vi "add logppms(SubVI).vi"(10 "字符串":string) -> (1 "ok or cancel":bool=TRUE, 2 "连接的字符串":string)   [LabVIEW 2019, in "SubVI.lvlib"]
uses:
  SubVI.lvlib
panel:
  in  "interval":dbl
  in  "cancel":bool
  in  "ok":bool
  in  "path":path
  in  "operation(0:open)":T1(ring)=enum."create"
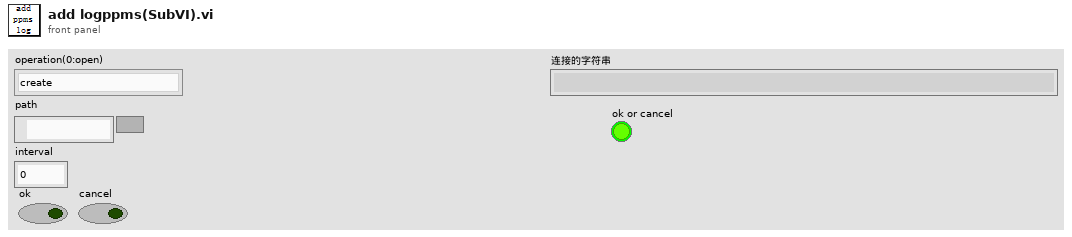
[diagram p1: front panel]
types:
  T1 = enum16{"open", "replace", "create", "open or create", "replace or create"}
  T2 = enum16{"open", "replace", "create", "open or create", "replace or create", "replace or create with confirmation"}
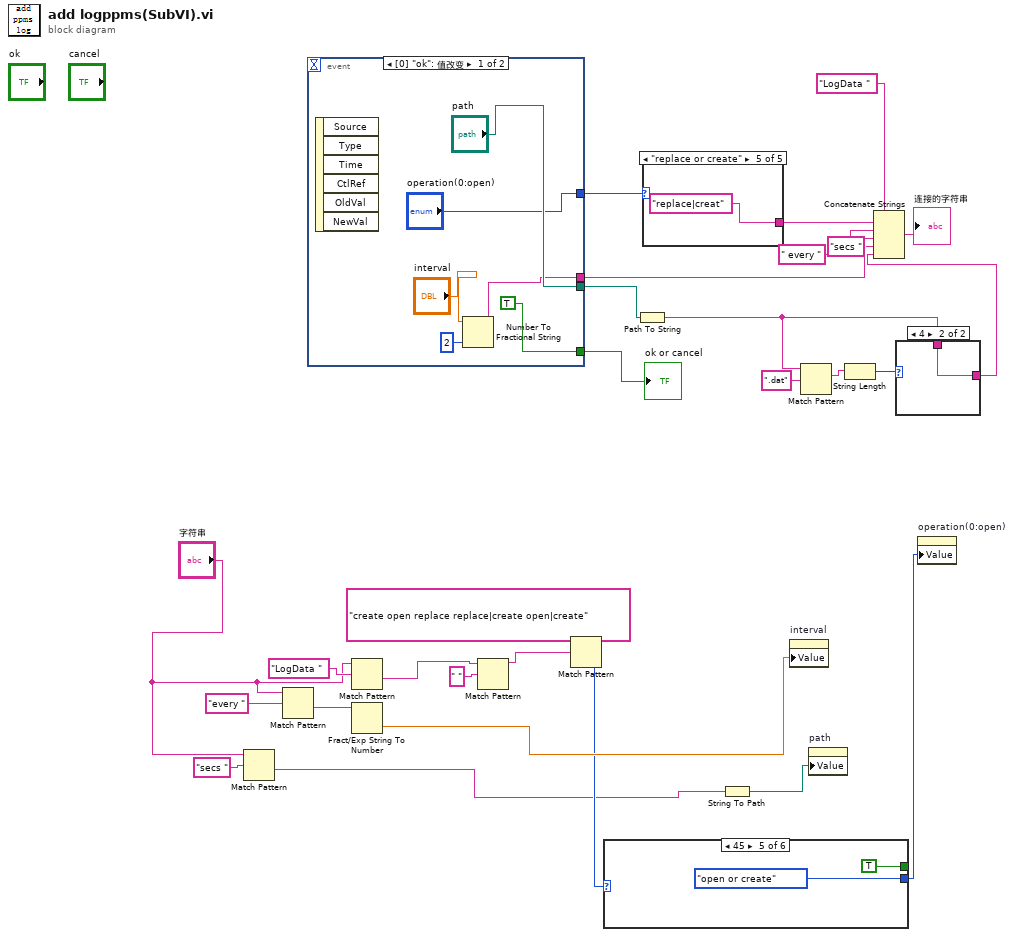
[diagram p0: block diagram]
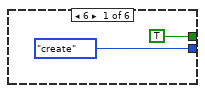
[diagram p2: hidden frame]
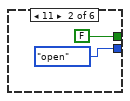
[diagram p3: hidden frame]
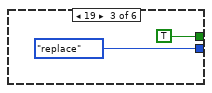
[diagram p4: hidden frame]
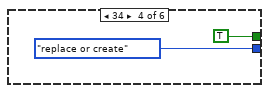
[diagram p5: hidden frame]
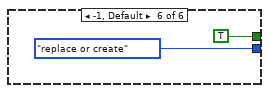
[diagram p6: hidden frame]
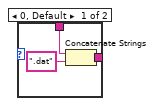
[diagram p7: hidden frame]
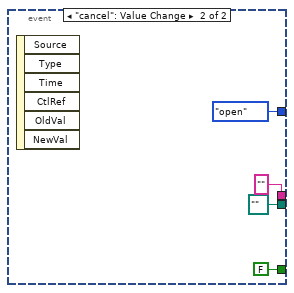
[diagram p8: hidden frame]
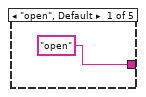
[diagram p9: hidden frame]
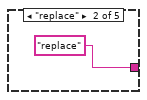
[diagram p10: hidden frame]
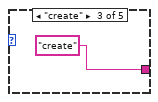
[diagram p11: hidden frame]
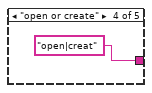
[diagram p12: hidden frame]
diagram:
  n1 = Match Pattern(string="字符串", regular expression="secs " ("正则表达式")) -> (after substring=w2:string)  [unwired: 1 in, 3 out]
  n2 = Match Pattern(string="字符串", regular expression="every " ("正则表达式")) -> (after substring=w11:string)  [unwired: 1 in, 3 out]
  n3 = event shown="[0] \"ok\": 值改变" {
    selector: _ -> [_ _]
    dyn-events: _ -> [_ _]
    timeout: _ -> [_ _]
    tunnel: ["path" path "" ("path")] -> w22
    tunnel: ["operation(0:open)" T1."open" ("operation(0:open)")] -> w27
    tunnel: [TRUE FALSE] -> w23
    tunnel: [w30 ""] -> w21
    event "ok": Value Change {
      n4 = event-data() -> ()  [unwired: 1 in, 6 out]
      n5 = Number To Fractional String(number="interval", precision (6)=i16 2 ("精度(6)")) -> (F-format string=w30:string)  [unwired: 2 in]
    }
    event "cancel": Value Change {
      n6 = event-data() -> ()  [unwired: 1 in, 6 out]
    }
  }
  "ok or cancel" <- w23
  n7 = Match Pattern(string="字符串", regular expression="LogData " ("正则表达式")) -> (after substring=w8:string)  [unwired: 1 in, 3 out]
  n8 = Fract/Exp String To Number(string=w11) -> (number=w5:dbl)  [unwired: 3 in, 1 out]
  n9 = Match Pattern(string=w8, regular expression=" " ("正则表达式")) -> (before substring=w7:string)  [unwired: 1 in, 3 out]
  n10 = Match Pattern(string="create open replace replace|create open|create" ("字符串"), regular expression=w7) -> (offset past match=w4:i32)  [unwired: 1 in, 3 out]
  n11 = case shown="45" w4 {
    tunnel: [T2."create" ("操作(0:open)") T2."open" ("操作(0:open)") T2."replace" ("操作(0:open)") T2."replace or create" ("操作(0:open)") T2."open or create" ("操作(0:open)") T2."replace or create" ("操作(0:open)")] -> w3
    tunnel: [TRUE FALSE TRUE TRUE TRUE TRUE] -> _
    frame 6 {
    }
    frame 11 {
    }
    frame 19 {
    }
    frame 34 {
    }
    frame 45 {
    }
    frame -1, Default {
    }
  }
  n12 = Path To String(path=w22) -> (string=w16:string)
  n13 = case shown="\"replace or create\"" w27 {
    tunnel: ["open" "replace" "create" "open|creat" "replace|creat"] -> w26
    frame "open", Default {
    }
    frame "replace" {
    }
    frame "create" {
    }
    frame "open or create" {
    }
    frame "replace or create" {
    }
  }
  n14 = String To Path(string=w2) -> (path=w1:path)
  n15 = property on="interval" class="DigNum (严格)"("Value"=w5) -> ()  [unwired: 2 in, 2 out]
  n16 = Match Pattern(string=w16, regular expression=".dat" ("正则表达式")) -> (match substring=w18:string)  [unwired: 1 in, 3 out]
  n17 = property on="path" class="Path"("Value"=w1) -> ()  [unwired: 2 in, 2 out]
  n18 = String Length(string=w18) -> (length=w17:i32)
  n19 = case shown="4" w17 {
    tunnel: w16 -> [w58 w59]
    tunnel: [w56 w59] -> w15
    frame 0, Default {
      n20 = Concatenate Strings(w58, ".dat" ("字符串")) -> (w56:string)
    }
    frame 4 {
    }
  }
  n21 = Concatenate Strings("LogData " ("字符串"), w26, " every " ("字符串"), w21, "secs " ("字符串"), w15) -> (→"连接的字符串":string)
  n22 = property on="operation(0:open)" class="Enum (严格)"("Value"=w3) -> ()  [unwired: 2 in, 2 out]
